vi "VICreate.vi"(0 "__args":cluster{"targetVi":string, "pattern":i32}) -> (1 "__return":i32, 2 "__errStatus":bool, 3 "__errCode":i32, 4 "__errSource":string)   [LabVIEW 2013]
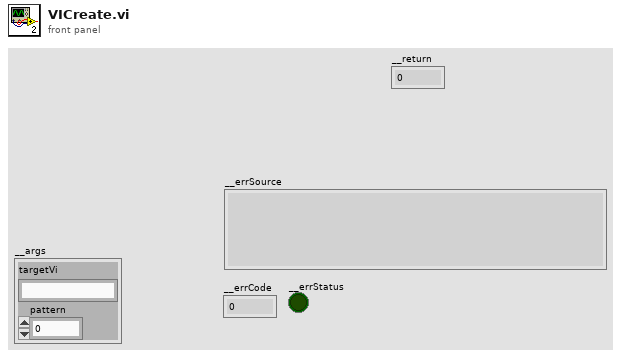
[diagram p1: front panel]
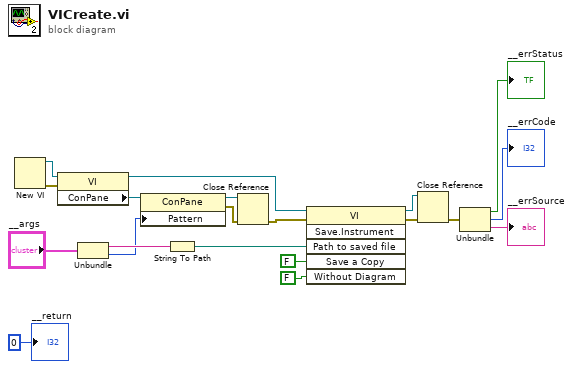
[diagram p0: block diagram]
diagram:
  n1 = New VI() -> (0:w6:errorcluster, 3:w8:refnum<vi>)  [unwired: 7 in]
  n2 = property class="VI"(reference=w8, error in=w6) -> (reference out=w7:refnum<vi>, "ConPane"=w5:refnum<vi>)  [unwired: 1 out]
  n3 = Unbundle("__args") -> ("targetVi"=w10:string, "pattern"=w1:i32)
  n4 = property class="ConPane"(reference=w5, "Pattern"=w1) -> (reference out=w3:refnum<vi>, error out=w2:errorcluster)  [unwired: 1 in]
  n5 = String To Path(string=w10) -> (path=w11:path)
  n6 = Close Reference(reference=w3, error in (no error)=w2) -> (error out=w4:errorcluster)
  n7 = invoke class="VI" method="Save.Instrument"(reference=w7, error in=w4, "Path to saved file"=w11, "Save a Copy"=FALSE, "Without Diagram"=FALSE) -> (reference out=w16:refnum<vi>, error out=w15:errorcluster)  [unwired: 1 in, 4 out]
  n8 = Close Reference(reference=w16, error in (no error)=w15) -> (error out=w12:errorcluster)
  n9 = Unbundle(w12) -> ("status"=→"__errStatus":bool, "code"=→"__errCode":i32, "source"=→"__errSource":string)
  "__return" <- 0
